vi "Initialize.vi"(8 "error in":errorcluster, 11 "Ballard ARINC 429 ref":T1 format="%.0x") -> (0 "error out":errorcluster, 3 "Ballard ARINC 429 ref out":T1 format="%.0x")   [LabVIEW 2020, in "AIM ARINC 429 System Explorer.lvlib" / "Implementation.lvlib"]
uses:
  Implementation.lvlib
  Scripting/AIM/AIM ARINC 429 Scripting.lvlib
  Shared/Initialization Method.ctl
  Shared/Device Parameters.ctl
  <vilib>/NI VeriStand/Custom Device API/Custom Device Item Ref.ctl
  <vilib>/NI VeriStand/Custom Device API/Custom Device API.lvlib
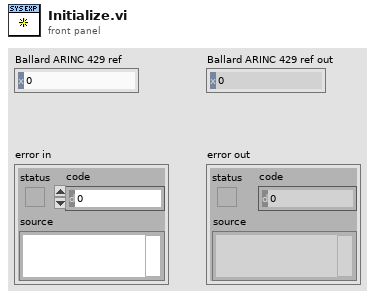
[diagram p1: front panel]
types:
  T1 = typedef "Custom Device API.lvlib/Custom Device Item Ref.ctl" = u64
  T2 = typedef "Device Parameters.ctl" = cluster{"initialization method":T3, "card number":i32, "PXI slot number":i32, "core number":i32}
  T3 = typedef "Initialization Method.ctl" = enum16{"PXI Slot Number", "Card Number"}
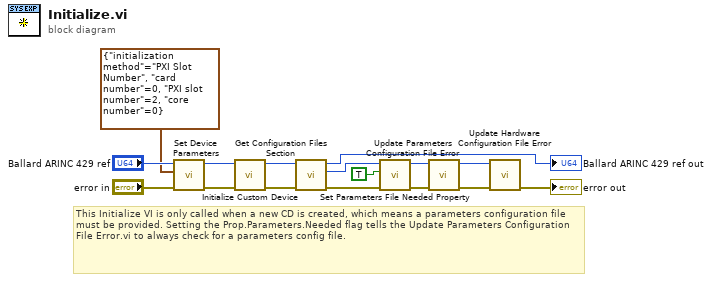
[diagram p0: block diagram]
diagram:
  # "This Initialize VI is only called when a new CD is created, which means a parameters configuration file must be provided. Setting the Prop.Parameters.Needed flag tells the Update Parameters Configuration File Error.vi to always check for a parameters config file."
  n1 = call "Set Device Parameters.vi"("error in"="error in", "device parameters"=T2 {"initialization method"=enum."PXI Slot Number", "card number"=0, "PXI slot number"=2, "core number"=0}, "Ballard ARINC 429 custom device in"="Ballard ARINC 429 ref") -> ("error out"=w7:errorcluster, "Ballard ARINC 429 custom device out"=w8:T1)  [unwired: 7 in]
  n2 = call "Initialize Custom Device.vi"("error in"=w7, "Ballard ARINC 429 ref"=w8) -> ("error out"=w5:errorcluster, "Ballard ARINC 429 ref out"=w4:T1)  [unwired: 8 in]
  n3 = call "Get Configuration Files Section.vi"("error in"=w5, "Custom device Ref"=w4) -> ("error out"=w2:errorcluster, "Configuration files Ref"=w6:T1, "Custom device Ref out"=→"Ballard ARINC 429 ref out":T1)  [unwired: 7 in]
  n4 = call "Set Parameters File Needed Property.vi"("error in"=w2, "needed"=TRUE, "configuration files ref"=w6) -> ("error out"=w16:errorcluster, "configuration files ref out"=w15:T1)  [unwired: 7 in]
  n5 = call "Update Parameters Configuration File Error.vi"("error in"=w16, "Configuration files Ref"=w15) -> ("error out"=w14:errorcluster, "Configuration files Ref out"=w12:T1)  [unwired: 8 in]
  n6 = call "Update Hardware Configuration File Error.vi"("error in"=w14, "Configuration files Ref"=w12) -> ("error out"=→"error out":errorcluster)  [unwired: 8 in, 1 out]
